vi "ToFTestertester.vi"(8 "error in":errorcluster, 9 "I2C Channel":u8=1, 11 "ToFs":T1[](array[typedef])=[enum."ToF1", enum."ToF2", enum."ToF3", enum."ToF5"]) -> (0 "error out":errorcluster, 1 "ToF Online":bool[](array[boolean]), 2 "ToF Details":T2[](array[typedef]) {"I2C Slave Address" format="%02x"})   [LabVIEW 2014]
uses:
  Sensors/Time of Flight - VL6180/VL6180 Resource.ctl
  Type Defs/Relays.ctl
panel:
  out "count":u8
  in  "wait (ms)":u32=150
  in  "Attempts":i32=2
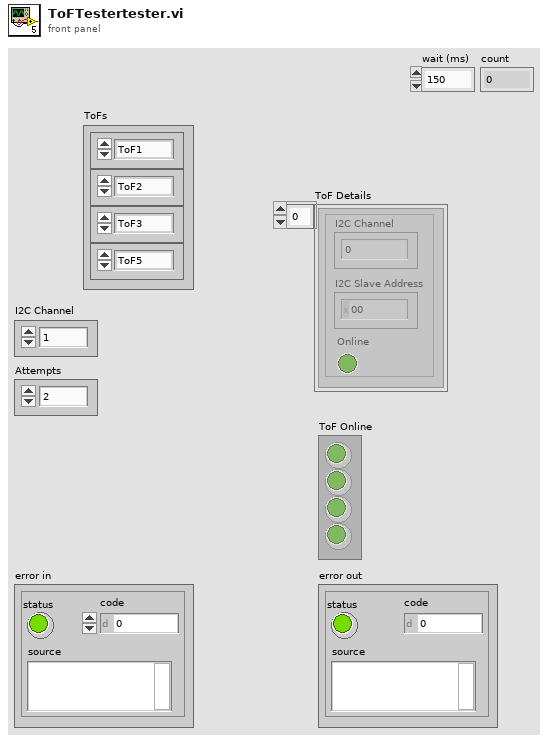
[diagram p1: front panel]
types:
  T1 = typedef "Relays.ctl" = enum16{"ToF1", "ToF2", "ToF3", "ToF4", "ToF5", "ToF6", "ToF7", "ToF8", "SensePwr", "All"}
  T2 = typedef "VL6180 Resource.ctl" = cluster{"I2C Channel":u8, "I2C Slave Address":u8, "Online":bool}
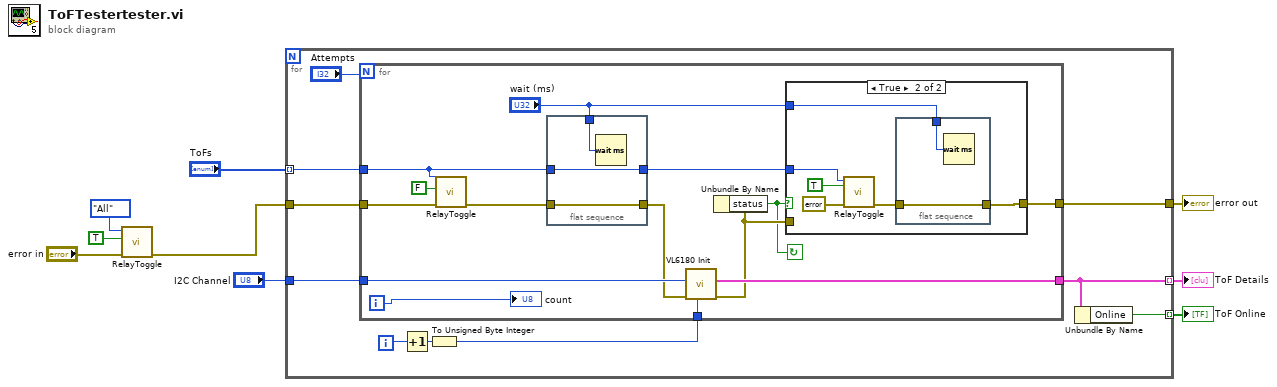
[diagram p0: block diagram]
diagram:
  n1 = call "RelayToggle.vi"("error in"="error in", "Power"=TRUE, "Relay"=Relays."All") -> ("error out"=w2:errorcluster)  [unwired: 8 in]
  n2 = for {
    tunnel: w2 -> [w19]
    tunnel: "I2C Channel" -> [w17]
    tunnel: [w11] -> w8
    tunnel: [w13] -> w7 mode=indexing
    tunnel: [w12] -> w6 mode=indexing
    tunnel: "ToFs" -> [w10] mode=indexing
    i -> [w18]
    n3 = Increment(x=w18) -> (x+1=w16:i32)
    n4 = To Unsigned Byte Integer(number=w16) -> (unsigned 8bit integer=w15:u8)
    n5 = for {
      N: "Attempts" -> [_]
      tunnel: w19 -> [w24]
      tunnel: w17 -> [w33]
      tunnel: w15 -> [w31]
      tunnel: [w30] -> w11
      tunnel: [w29] -> w13
      tunnel: w10 -> [w21]
      i -> [w27]
      stop <- w25 continue-if-true
      n6 = call "RelayToggle.vi"("error in"=w24, "Power"=FALSE, "Relay"=w21) -> ("error out"=w23:errorcluster)  [unwired: 8 in]
      n7 = flat-sequence {
        tunnel: [w45] -> w32
        tunnel: w23 -> [w45]
        tunnel: "wait (ms)" -> [w44]
        tunnel: w21 -> [w43]
        tunnel: [w43] -> w20
        frame #0 {
          n8 = Wait (ms)(milliseconds to wait=w44) -> ()  [unwired: 1 out]
        }
      }
      n9 = call "VL6180 Init.vi"("Change Slave Address"=w31, "Error In"=w32, "I2C Channel"=w33) -> ("Error Out"=w26:errorcluster, "VL6180 Resource"=w29:T2)  [unwired: 6 in, 1 out]
      n10 = Unbundle By Name(w26) -> ("status"=w25:bool)
      n11 = case shown="True" w25 {
        tunnel: [w34 w37] -> w30
        tunnel: "wait (ms)" -> [_ w40]
        tunnel: w26 -> [w34 _]
        tunnel: w20 -> [_ w35]
        frame False {
        }
        frame True {
          n12 = call "RelayToggle.vi"("error in"=errorcluster {"status"=FALSE, "code"=0, "source"=""} ("error in (no error)"), "Power"=TRUE, "Relay"=w35) -> ("error out"=w36:errorcluster)  [unwired: 8 in]
          n13 = flat-sequence {
            tunnel: w40 -> [w42]
            tunnel: [w41] -> w37
            tunnel: w36 -> [w41]
            frame #0 {
              n14 = Wait (ms)(milliseconds to wait=w42) -> ()  [unwired: 1 out]
            }
          }
        }
      }
      "count" <- w27
    }
    n15 = Unbundle By Name(w13) -> ("Online"=w12:bool)
  }
  "error out" <- w8
  "ToF Details" <- w7
  "ToF Online" <- w6
